vi "Save Processed Via.vi"(4 "Output Folder":path, 6 "Output File":path, 8 "error in (no error)":errorcluster, 10 "Processed Via":string, 11 "GVIWebProcessorApp in":refnum<class "GVIWebProcessorApp.lvclass">) -> (0 "error out":errorcluster, 3 "GVIWebProcessorApp out":refnum<class "GVIWebProcessorApp.lvclass">)   [LabVIEW 2020, in "PicoG-Processor.lvlib" / "GVIWebProcessorApp.lvclass"]
uses:
  GVIWebProcessorApp.lvclass
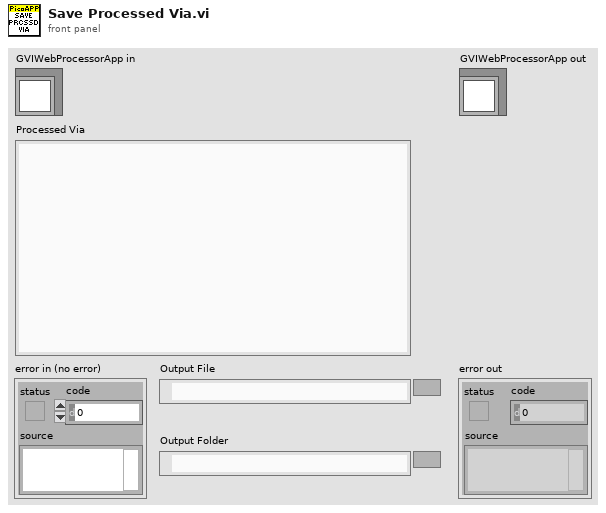
[diagram p1: front panel]
types:
  T1 = enum16{"open", "replace", "create", "open or create", "replace or create", "replace or create with confirmation"}
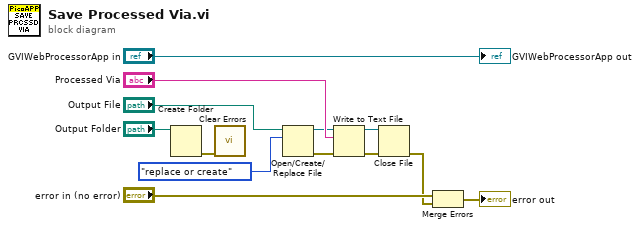
[diagram p0: block diagram]
diagram:
  n1 = Create Folder(path (use dialog)="Output Folder") -> (error out=w10:errorcluster)  [unwired: 2 in, 2 out]
  n2 = call <vilib>:"Clear Errors.vi"("error in (no error)"=w10) -> ()  [unwired: 5 in, 2 out]
  n3 = Open/Create/Replace File(file path (use dialog)="Output File", operation (0:open)=T1."replace or create") -> (refnum out=w3:refnum<file>, error out=w4:errorcluster)  [unwired: 4 in, 1 out]
  n4 = Write to Text File(file (use dialog)=w3, text="Processed Via", error in=w4) -> (refnum out=w7:refnum<file>, error out=w8:errorcluster)  [unwired: 1 in, 1 out]
  n5 = Close File(refnum=w7, error in=w8) -> (error out=w5:errorcluster)  [unwired: 1 out]
  n6 = Merge Errors("error in (no error)", w5) -> (→"error out":errorcluster)
  "GVIWebProcessorApp out" <- "GVIWebProcessorApp in"
